vi "Initialize.vi"(8 "error in (no error)":errorcluster, 9 "Timeout (2500ms)":i32=2500, 10 "Port (4223)":u16=4223, 11 "IP (localhost)":string="localhost") -> (0 "error out":errorcluster, 3 "IP Connection out":refnum<class "IP Connection.lvclass">)   [LabVIEW 2011, in "Tinkerforge.lvlib" / "IP Connection.lvclass"]
doc: "This VI initializes a <B>IP Connction</B> class object. It connects to the Brickd and calls the communication worker VI."
uses:
  IP Connection.lvclass
  Type Definitions/Errors.ctl
  Type Definitions/Connection Status.ctl
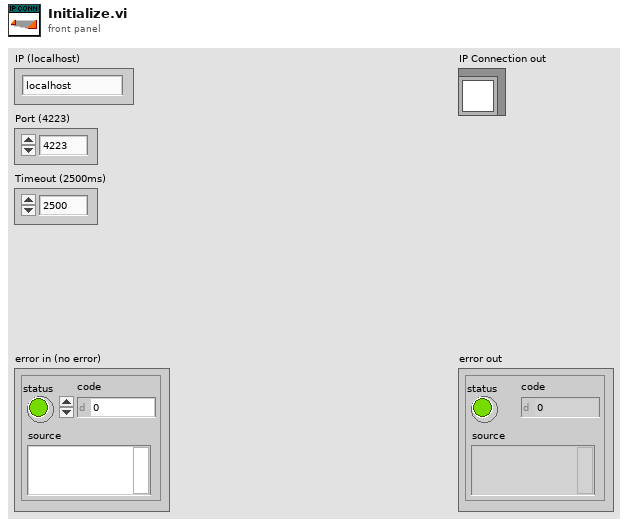
[diagram p1: front panel]
types:
  T1 = typedef "Tinkerforge.lvlib/IP Connection.lvclass/Connection Status.ctl" = enum16{"Uninitialized", "Connected", "Reconnecting", "Disconnected"}
  T2 = typedef "Tinkerforge.lvlib/IP Connection.lvclass/Errors.ctl" = enum16{"Timeout", "Device type incorrect", "Device already added", "Device not existing"}
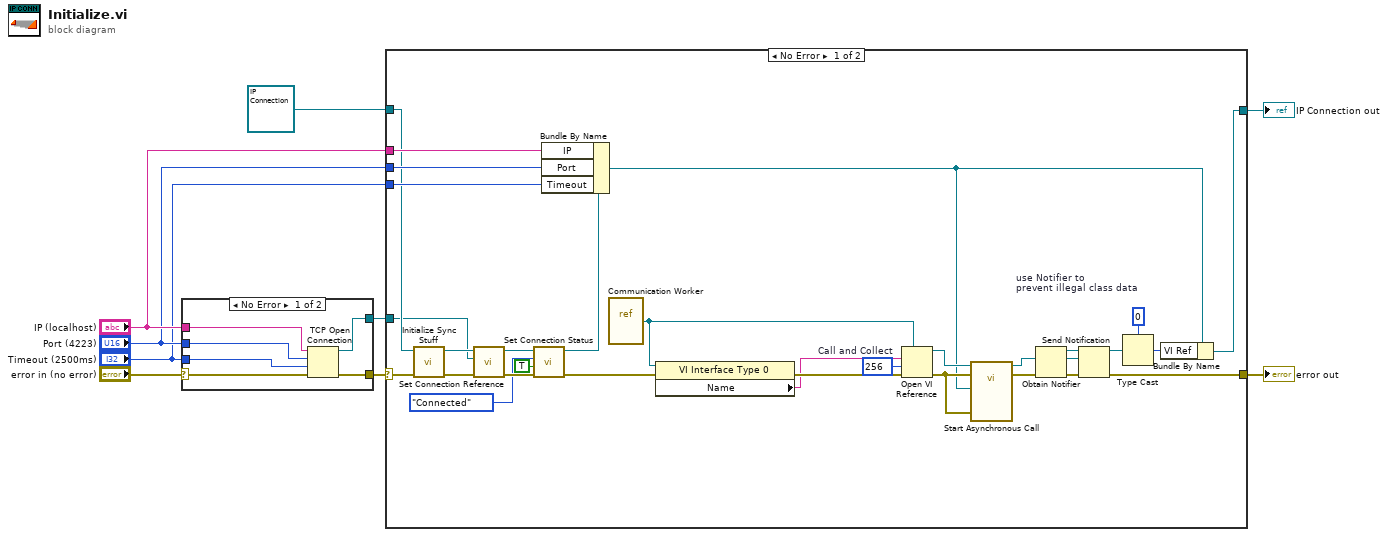
[diagram p0: block diagram]
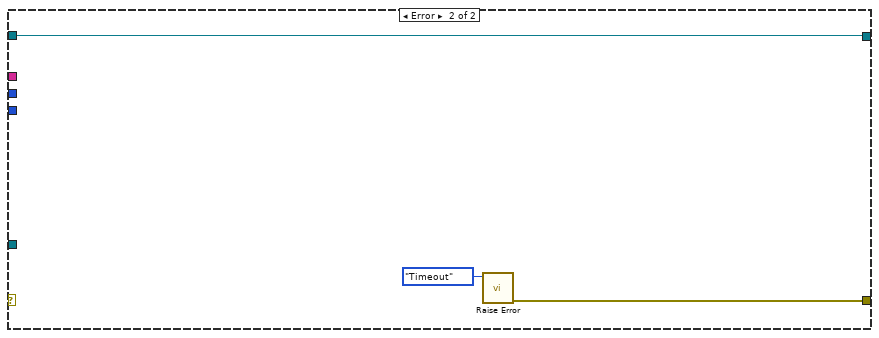
[diagram p2: hidden frame]
diagram:
  n1 = case shown="No Error" "error in (no error)" {
    selector: "error in (no error)" -> [w15 w16]
    tunnel: [w14 w16] -> w1
    tunnel: "IP (localhost)" -> [w13 _]
    tunnel: "Port (4223)" -> [w12 _]
    tunnel: "Timeout (2500ms)" -> [w11 _]
    tunnel: [w10 _] -> w4
    frame No Error {
      n2 = TCP Open Connection(address=w13, remote port or service name=w12, timeout ms (60000)=w11, error in (no error)=w15) -> (connection ID=w10:refnum<k5>, error out=w14:errorcluster)  [unwired: 1 in]
    }
    frame Error {
    }
  }
  n3 = case shown="No Error" w1 {
    selector: w1 -> [w30 _]
    tunnel: [w27 w48] -> w8
    tunnel: "IP (localhost)" -> [w46 _]
    tunnel: "Port (4223)" -> [w45 _]
    tunnel: "Timeout (2500ms)" -> [w44 _]
    tunnel: refnum<class "IP Connection.lvclass"> refnum ("Tinkerforge.lvlib:IP Connection.lvclass") -> [w29 w49]
    tunnel: w4 -> [w23 _]
    tunnel: [w28 w49] -> w3
    frame No Error {
      w32 = u32 0  # use Notifier to prevent illegal class data
      w43 = 256  # Call and Collect
      n4 = call "Initialize Sync Stuff.vi"("error in (no error)"=w30, "IP Connection in"=w29) -> ("error out"=w25:errorcluster, "IP Connection out"=w24:refnum<class "IP Connection.lvclass">)  [unwired: 8 in]
      n5 = call "Set Connection Reference.vi"("error in (no error)"=w25, "TCP Network Connection"=w23, "IP Connection in"=w24) -> ("error out"=w22:errorcluster, "IP Connection out"=w21:refnum<class "IP Connection.lvclass">)  [unwired: 7 in]
      n6 = call "Set Connection Status.vi"("error in (no error)"=w22, "connected?"=TRUE, "Connection Status"=Connection_Status."Connected", "IP Connection in"=w21) -> ("error out"=w20:errorcluster, "IP Connection out"=w19:refnum<class "IP Connection.lvclass">)  [unwired: 6 in]
      n7 = Bundle By Name(cluster=w19, "IP"=w46, "Port"=w45, "Timeout"=w44) -> (w37:refnum<class "IP Connection.lvclass">)
      n8 = vi-ref "Communication Worker.vi"() -> (w38:refnum<vi>)
      n9 = property class="VI Interface Type 0"(reference=w38, error in=w20) -> (error out=w40:errorcluster, "Name"=w39:string)  [unwired: 1 out]
      n10 = Open VI Reference(type specifier VI Refnum (for type only)=w38, vi path=w39, options=w43, error in (no error)=w40) -> (vi reference=w42:refnum<vi>, error out=w41:errorcluster)  [unwired: 2 in]
      n11 = call-by-ref "Start Asynchronous Call"(reference=w42, error in=w41, 8:"error in (no error)"=w41, "IP Connection in"=w37) -> (reference out=w26:refnum<vi>, error out=w36:errorcluster)  [unwired: 8 in, 2 out]
      n12 = Obtain Notifier(notification data type=w26, error in (no error)=w36) -> (notifier out=w34:refnum<notifier>, error out=w35:errorcluster)  [unwired: 2 in, 1 out]
      n13 = Send Notification(notification=w26, notifier=w34, error in (no error)=w35) -> (notifier out=w33:refnum<notifier>, error out=w27:errorcluster)
      n14 = Type Cast(type=w32, x=w33) -> (*(type *) &x=w31:u32)
      n15 = Bundle By Name(cluster=w37, "VI Ref"=w31) -> (w28:refnum<class "IP Connection.lvclass">)
    }
    frame Error {
      n16 = call "Raise Error.vi"("Error"=Errors."Timeout") -> ("Error Out"=w48:errorcluster)  [unwired: 10 in]
    }
  }
  "error out" <- w8
  "IP Connection out" <- w3
